vi "TeleOp_TwistCalc.vi"(10 "Slow Button":bool, 11 "Input Twist":dbl) -> (3 "Output Twist":dbl)   [LabVIEW 2017]
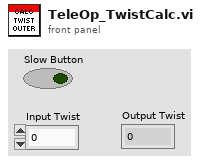
[diagram p1: front panel]
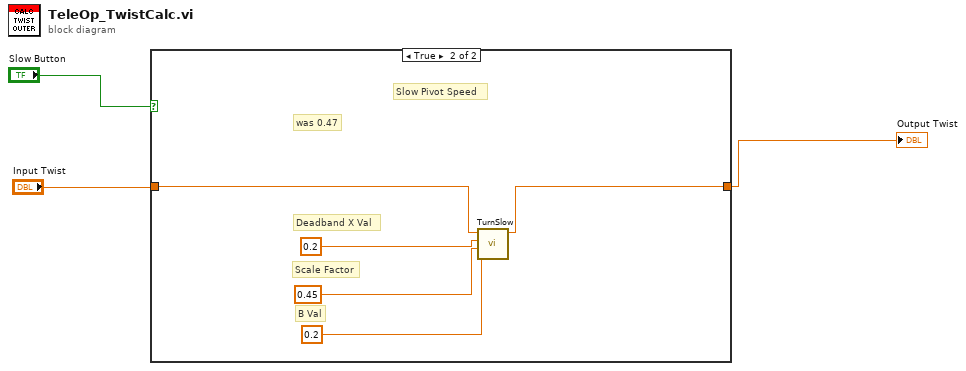
[diagram p0: block diagram]
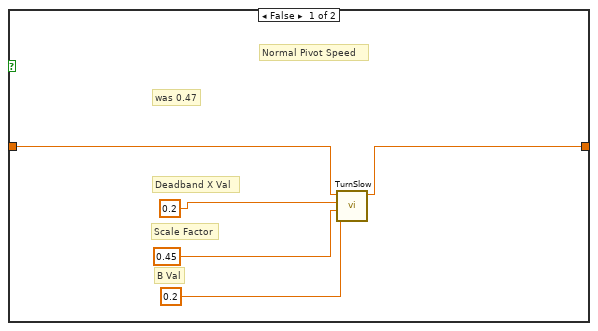
[diagram p2: hidden frame]
diagram:
  n1 = case shown="True" "Slow Button" {
    tunnel: "Input Twist" -> [w6 w13]
    tunnel: [w5 w12] -> w1
    frame False {
      # "was 0.47"
      # "B Val"
      # "Scale Factor"
      # "Deadband X Val"
      # "Normal Pivot Speed"
      n2 = call "TurnSlow.vi"("b - value"=0.2 ("b value"), "Scale Factor"=0.45, "Deadband X value"=0.2, "Input Twist"=w6) -> ("Twist Output"=w5:dbl)  [unwired: 7 in]
    }
    frame True {
      # "was 0.47"
      # "B Val"
      # "Scale Factor"
      # "Deadband X Val"
      # "Slow Pivot Speed"
      n3 = call "TurnSlow.vi"("b - value"=0.2 ("b value"), "Scale Factor"=0.45, "Deadband X value"=0.2, "Input Twist"=w13) -> ("Twist Output"=w12:dbl)  [unwired: 7 in]
    }
  }
  "Output Twist" <- w1
